vi "Camera Popup Settings.vi"(8 "error in (no error)":errorcluster, 9 "Configuration":T1={"Settings"={"Pixel clock"=20, "Frame rate"=30.0, "Exposure time"=33.21525, "Master Gain"=0, "Red Gain"=0, "Green Gain"=0, "Blue Gain"=0, "Auto Gain"=FALSE, "White-balance"=FALSE, "Color Correction"=FALSE}} {"Settings"."Blue Gain" min=0 max=100 scale=0.0..100.0; "Settings"."Green Gain" min=0 max=100 scale=0.0..100.0; "Settings"."Red Gain" min=0 max=100 scale=0.0..100.0; "Settings"."Master Gain" min=0 max=100 scale=0.0..100.0; "Settings"."Exposure time" min=0.101625 max=159.246375 step=0.101625 scale=0.101625..159.246375 scale format="%#.3g"; "Settings"."Frame rate" min=2.7455631699174137 max=6.2675785993528725 step=0.000101625 scale=2.7455631699174137..6.2675785993528725 scale format="%^#_3g"; "Settings"."Pixel clock" min=5 max=43 scale=5.0..43.0}, 10 "Camera":refnum<queue>, 11 "Function":enum16{"Initialize", "Action"}(ring)) -> (0 "error out":errorcluster)   [LabVIEW 2014]
uses:
  Camera Config.ctl
  Camera Settings.ctl
  support/Message Queue/Message Cluster.ctl
  support/Message Queue/Message Queue.lvlib
panel:
  in  "Master Gain":i32(slide) min=0 max=100 step=1 scale=0.0..100.0
  in  "Exposure time":dbl(slide)=33.21525 min=0.101625 max=159.246375 step=0.271 scale=0.271..424.65700000000004 scale format="%#.3g"
  # "LICENSED MATERIALS – PROPERTY OF IBM\nCopyright IBM Corp. 2016,\nALL RIGHTS RESERVED"
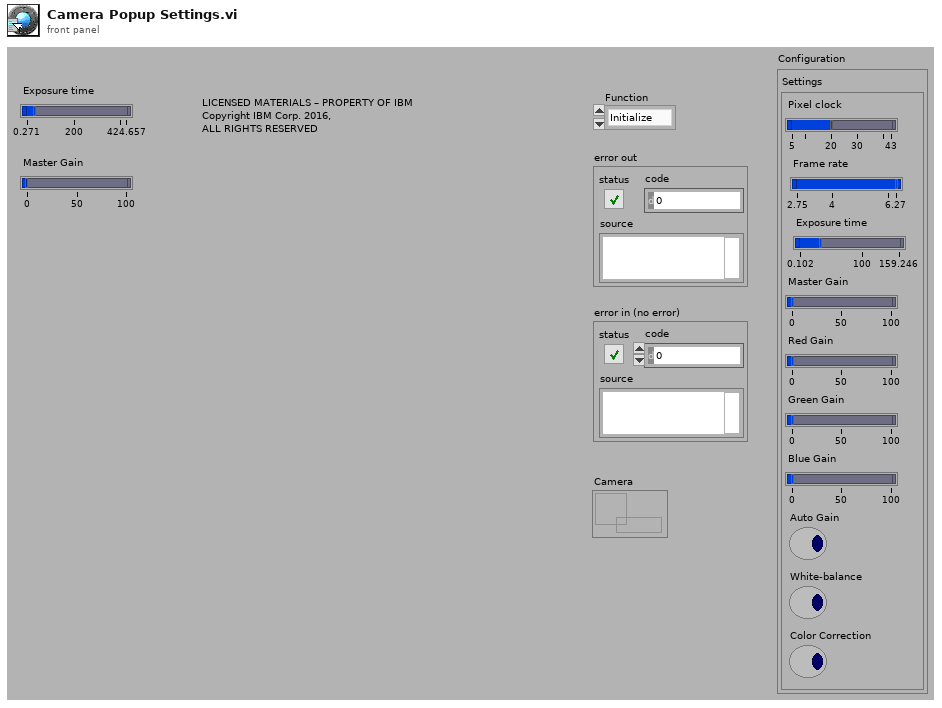
[diagram p1: front panel]
types:
  T1 = typedef "Camera Config.ctl" = cluster{"Settings":T2}
  T2 = typedef "Camera Settings.ctl" = cluster{"Pixel clock":i32, "Frame rate":dbl, "Exposure time":dbl, "Master Gain":i32, "Red Gain":i32, "Green Gain":i32, "Blue Gain":i32, "Auto Gain":bool, "White-balance":bool, "Color Correction":bool}
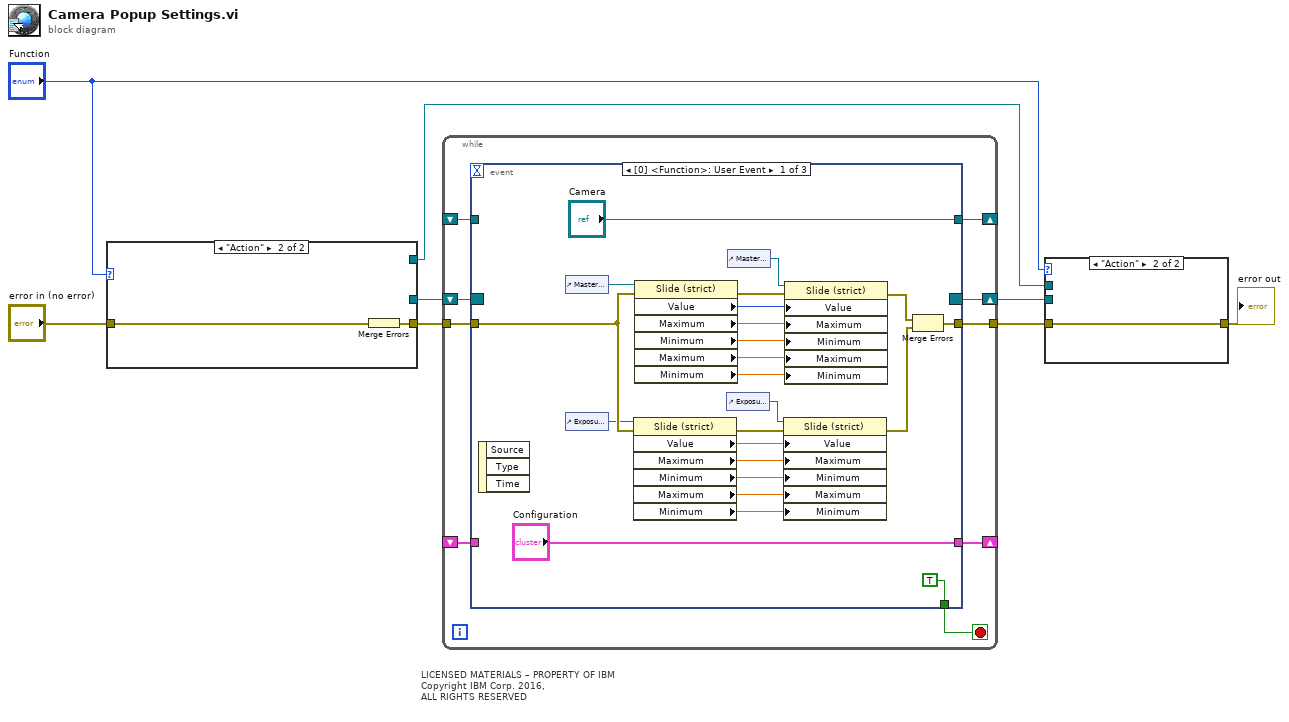
[diagram p0: block diagram]
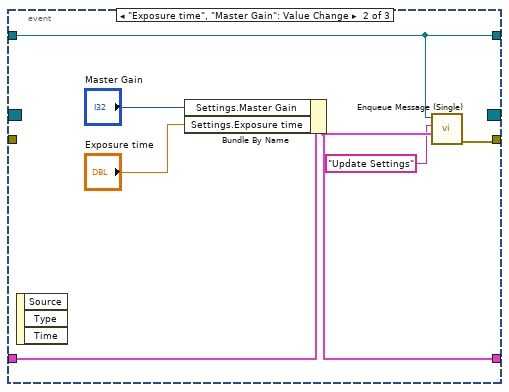
[diagram p2: hidden frame]
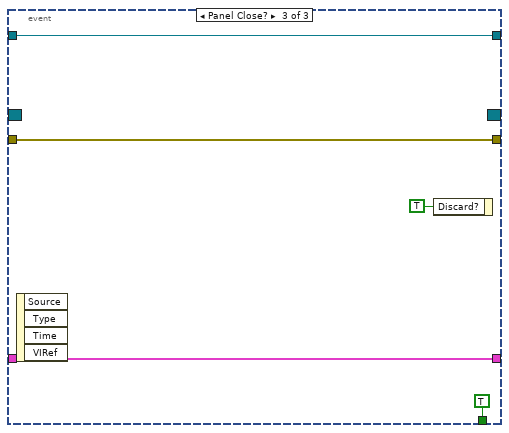
[diagram p3: hidden frame]
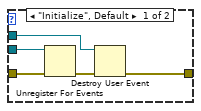
[diagram p4: hidden frame]
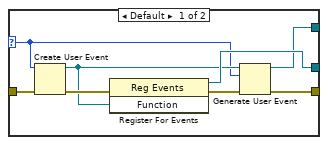
[diagram p5: hidden frame]
diagram:
  # "LICENSED MATERIALS – PROPERTY OF IBM\nCopyright IBM Corp. 2016,\nALL RIGHTS RESERVED"
  n1 = case shown="\"Action\"" "Function" {
    selector: "Function" -> [w11 _]
    tunnel: [w16 _] -> w4
    tunnel: [w9 w18] -> w1
    tunnel: "error in (no error)" -> [w10 w17]
    tunnel: [w12 _] -> w5
    frame Default {
      n2 = Create User Event(user event datatype=w11, error in=w10) -> (user event=w14:refnum<user-event>, error out=w15:errorcluster)
      n3 = register-events(error in=w15, w14) -> (reference out=w16:refnum<event-registration>, error out=w13:errorcluster)  [unwired: 1 in]
      n4 = Generate User Event(user event=w14, event data cluster=w11, error in=w13) -> (user event out=w12:refnum<user-event>, error out=w9:errorcluster)  [unwired: 1 in]
    }
    frame "Action" {
      n5 = Merge Errors(w17) -> (w18:errorcluster)
    }
  }
  n6 = while {
    shift-right: [w26] -> w3
    shift-left: w4 -> [w27]
    shift-right: [w25] -> _
    shift-left: _ -> [w24]
    shift-right: [w23] -> _
    shift-left: _ -> [w22]
    tunnel: [w21] -> w2
    tunnel: w1 -> [w20]
    stop <- w19 stop-if-true
    n7 = event shown="[0] <Function>: User Event" {
      selector: w27 -> [_ _ _]
      dyn-events: [_ _ _] -> w26
      timeout: _ -> [_ _ _]
      tunnel: ["Configuration" w52 w62] -> w23
      tunnel: ["Camera" w56 w61] -> w25
      tunnel: w24 -> [_ w56 w61]
      tunnel: w22 -> [_ w53 w62]
      tunnel: [w33 w57 w59] -> w21
      tunnel: w20 -> [w35 _ w59]
      tunnel: [TRUE _ TRUE] -> w19
      event User Event {
        n8 = event-data() -> ()  [unwired: 1 in, 3 out]
        n9 = control-ref of="Master Gain"() -> (w31:refnum<vi>)
        n10 = control-ref of="Exposure time"() -> (w30:refnum<vi>)
        n11 = property on="Property Node" class="Slide (strict)"(reference=w30, error in=w35) -> (error out=w46:errorcluster, "Value"=w40:dbl, "Maximum"=w39:dbl, "Minimum"=w38:dbl, "Maximum"=w37:dbl, "Minimum"=w36:dbl)  [unwired: 1 out]
        n12 = property on="Property Node" class="Slide (strict)"(reference=w31, error in=w35) -> (error out=w47:errorcluster, "Value"=w45:i32, "Maximum"=w44:dbl, "Minimum"=w43:dbl, "Maximum"=w42:dbl, "Minimum"=w41:dbl)  [unwired: 1 out]
        n13 = control-ref of="Exposure time"() -> (w29:refnum<vi>)
        n14 = control-ref of="Master Gain"() -> (w28:refnum<vi>)
        n15 = property on="Property Node" class="Slide (strict)"(reference=w29, error in=w46, "Value"=w40, "Maximum"=w39, "Minimum"=w38, "Maximum"=w37, "Minimum"=w36) -> (error out=w32:errorcluster)  [unwired: 1 out]
        n16 = property on="Property Node" class="Slide (strict)"(reference=w28, error in=w47, "Value"=w45, "Maximum"=w44, "Minimum"=w43, "Maximum"=w42, "Minimum"=w41) -> (error out=w34:errorcluster)  [unwired: 1 out]
        n17 = Merge Errors(w34, w32) -> (w33:errorcluster)
      }
      event "Exposure time", "Master Gain": Value Change {
        n18 = event-data() -> ()  [unwired: 1 in, 3 out]
        n19 = Bundle By Name(cluster=w53, "Settings.Master Gain"="Master Gain", "Settings.Exposure time"="Exposure time") -> (w52:T1)
        n20 = call "Enqueue Message (Single).vi"("Message Data"=w52, "Message"="Update Settings", "Message Queue"=w56) -> ("error out"=w57:errorcluster)  [unwired: 1 in, 7 out]
      }
      event Panel Close? {
        n21 = event-data() -> ()  [unwired: 1 in, 4 out]
        n22 = event-data("Discard?"=TRUE) -> ()  [unwired: 1 in, 1 out]
      }
    }
  }
  n23 = case shown="\"Action\"" "Function" {
    tunnel: w2 -> [w67 w68]
    tunnel: [w64 w68] -> w7
    tunnel: w3 -> [w65 _]
    tunnel: w5 -> [w63 _]
    frame "Initialize", Default {
      n24 = Unregister For Events(event registration refnum=w65, error in=w67) -> (error out=w66:errorcluster)
      n25 = Destroy User Event(user event=w63, error in=w66) -> (error out=w64:errorcluster)
    }
    frame "Action" {
    }
  }
  "error out" <- w7
